vi "main_web_run_as_admin.vi"   [LabVIEW 2015, in "lv-hello-world.lvlib"]
uses:
  lv-hello-world.lvlib
  <userlib>/antonio-alexander/lv-bin-windows/public/api/v1/v1.lvlib
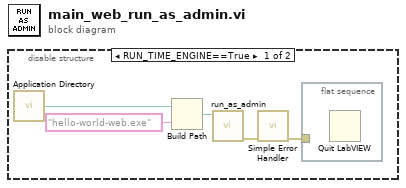
[diagram p0: block diagram]
diagram:
  n1 = disable-structure shown="RUN_TIME_ENGINE==True" {
    frame condition #0 {
      n2 = call <vilib>:"Application Directory.vi"() -> ("Application Directory"=w5:path)
      n3 = Build Path(base path=w5, name or relative path="hello-world-web.exe") -> (appended path=w4:path)
      n4 = call <userlib>:"run_as_admin.vi"("command"=w4) -> ("error out"=w3:errorcluster)  [unwired: 10 in]
      n5 = call <vilib>:"Simple Error Handler.vi"("error in (no error)"=w3) -> ("error out"=w1:errorcluster)  [unwired: 4 in, 4 out]
      n6 = flat-sequence {
        tunnel: w1 -> [_]
        frame #0 {
          n7 = Quit LabVIEW() -> ()  [unwired: 1 in]
        }
      }
    }
    frame condition #1 (active) {
    }
  }
